vi "Adjust Min-Max.vi"(7 "log?":bool, 8 "error in (no error)":errorcluster, 9 "Secondary Graph":refnum<vi>, 10 "Primary Graph":refnum<vi>, 11 "Scan Driver.lvclass":refnum<class "Scan Driver.lvclass">) -> (0 "error out":errorcluster, 2 "High":dbl, 3 "Scan Driver.lvclass out":refnum<class "Scan Driver.lvclass">)   [LabVIEW 2009, in "Scan Driver.lvclass"]
doc: "Set the boundaries of the onscreen scan graphs according to the extrema of the data store."
uses:
  Scan Driver.lvclass
  Scan Driver.lvclass/Scan Driver.ctl
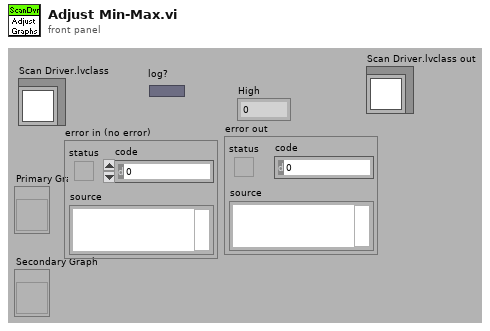
[diagram p1: front panel]
types:
  T1 = typedef "Readable.lvclass/Data Point.ctl" = dbl
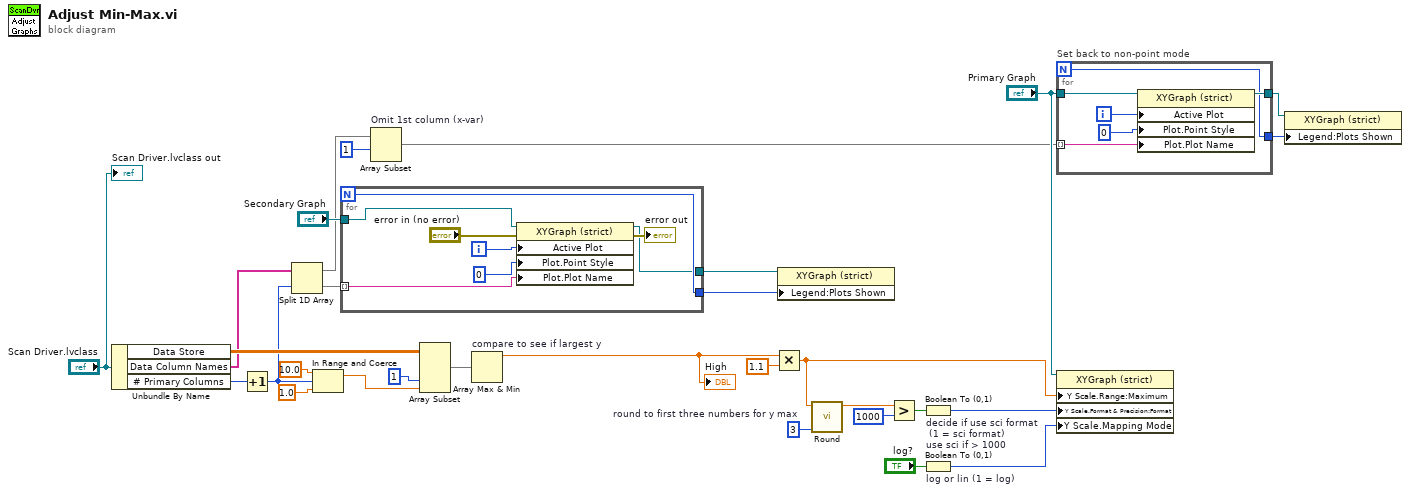
[diagram p0: block diagram]
diagram:
  w15 = 3  # round to first three numbers for y max
  n1 = Unbundle By Name("Scan Driver.lvclass") -> ("Data Store"=w20:T1[][], "Data Column Names"=w10:string[], "# Primary Columns"=w12:u32)
  n2 = Increment(x=w12) -> (x+1=w11:u32)
  n3 = Split 1D Array(array=w10, index=w11) -> (first subarray=w8:string[], second subarray=w9:string[])
  n4 = In Range and Coerce(upper limit=10.0, x=w11, lower limit=1.0) -> (coerced(x)=w18:dbl)  [unwired: 1 out]
  n5 = for {
    N -> [w32]
    tunnel: "Secondary Graph" -> [w37]
    tunnel: w9 -> [w33] mode=indexing
    tunnel: [w32] -> w4
    tunnel: [w31] -> w3
    i -> [w38]
    n6 = property on="Property Node" class="XYGraph (strict)"(reference=w37, error in="error in (no error)", "Active Plot"=w38, "Plot.Point Style"=0, "Plot.Plot Name"=w33) -> (reference out=w31:refnum<vi>, error out=→"error out":errorcluster)
  }
  n7 = Array Subset "Omit 1st column (x-var)"(array=w8, index=1) -> (w6:string[])  [unwired: 1 in]
  n8 = Array Subset(array=w20, index (col)=1, length (col)=w18) -> (w5:T1[][])  [unwired: 2 in]
  n9 = Array Max & Min "compare to see if largest y"(array=w5) -> (max value=w30:T1)  [unwired: 3 out]
  "High" <- w30
  n10 = Multiply(x=w30, y=1.1) -> (x*y=w14:T1)
  n11 = property on="Property Node" class="XYGraph (strict)"(reference=w3, "Legend:Plots Shown"=w4) -> ()  [unwired: 1 in, 2 out]
  n12 = call "Round.vi"("place at this power of 10"=w15, "Number In"=w14) -> ("Number Out"=w13:dbl)  [unwired: 5 out]
  n13 = Greater?(x=w13, y=1000) -> (0:w24:bool)
  n14 = Boolean To (0,1) "decide if use sci format\n (1 = sci format)\nuse sci if > 1000"(Boolean=w24) -> (0, 1=w25:i16)
  n15 = Boolean To (0,1) "log or lin (1 = log)"(Boolean="log?") -> (0, 1=w26:i16)
  n16 = for "Set back to non-point mode" {
    N -> [w39]
    tunnel: "Primary Graph" -> [w43]
    tunnel: w6 -> [w41] mode=indexing
    tunnel: [w40] -> w2
    tunnel: [w39] -> w1
    i -> [w44]
    n17 = property on="Property Node" class="XYGraph (strict)"(reference=w43, "Active Plot"=w44, "Plot.Point Style"=0, "Plot.Plot Name"=w41) -> (reference out=w40:refnum<vi>)  [unwired: 1 in, 1 out]
  }
  n18 = property on="Property Node" class="XYGraph (strict)"(reference="Primary Graph", "Y Scale.Range:Maximum"=w14, "Y Scale.Format & Precision:Format"=w25, "Y Scale.Mapping Mode"=w26) -> ()  [unwired: 1 in, 2 out]
  n19 = property on="Property Node" class="XYGraph (strict)"(reference=w2, "Legend:Plots Shown"=w1) -> ()  [unwired: 1 in, 2 out]
  "Scan Driver.lvclass out" <- "Scan Driver.lvclass"
